vi "ValidateResults.vi"(8 "start_icfft":i32, 9 "PowerSpectrum":dbl[][](array[numeric]), 10 "Array of Power\nSpectrum Data":T1[](array[typedef]), 11 "Max Error":dbl) -> (2 "Boolean":bool, 3 "Max Error":dbl[](array[numeric]))   [LabVIEW 2015, in "SETI_LV.lvlib"]
uses:
  TypeDefs/Power Spectrum Data.ctl
  SETI_LV.lvlib
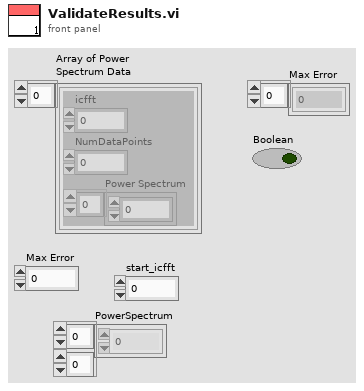
[diagram p1: front panel]
types:
  T1 = typedef "SETI_LV.lvlib/Power Spectrum Data.ctl" = cluster{"icfft":i32, "NumDataPoints":i32, "Power Spectrum":sgl[]}
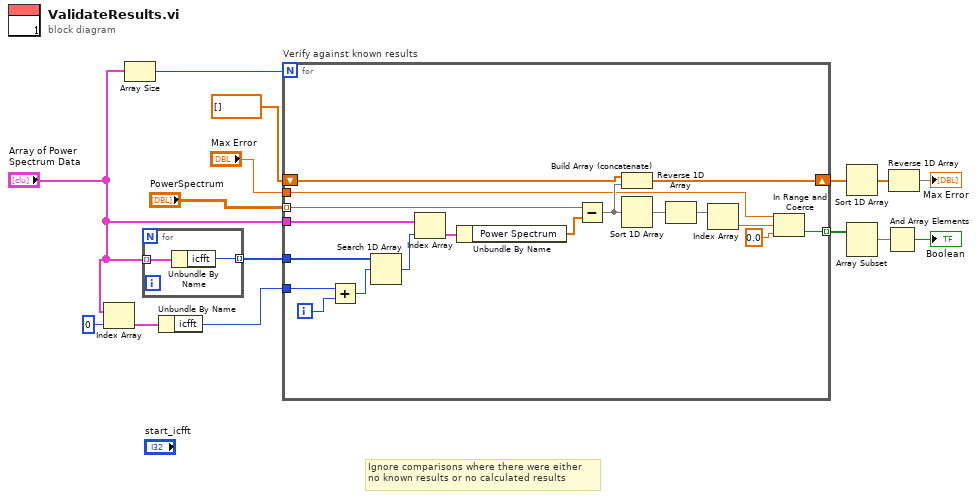
[diagram p0: block diagram]
diagram:
  # "Ignore comparisons where there were either\nno known results or no calculated results"
  n1 = Index Array(array="Array of Power\nSpectrum Data", index=0) -> (element=w2:T1)
  n2 = Array Size(array="Array of Power\nSpectrum Data") -> (size(s)=w5:i32)
  n3 = for {
    tunnel: "Array of Power\nSpectrum Data" -> [w17] mode=indexing
    tunnel: [w16] -> w9 mode=indexing
    n4 = Unbundle By Name(w17) -> ("icfft"=w16:i32)
  }
  n5 = Unbundle By Name(w2) -> ("icfft"=w1:i32)
  n6 = for "Verify against known results" {
    N: w5 -> [_]
    tunnel: "PowerSpectrum" -> [w23] mode=indexing
    tunnel: w1 -> [w34]
    tunnel: w9 -> [w31]
    tunnel: [w24] -> w10 mode=indexing
    tunnel: "Array of Power\nSpectrum Data" -> [w19]
    shift-right: [w21] -> w12
    shift-left: dbl[] [] -> [w20]
    tunnel: "Max Error" -> [w18]
    i -> [w33]
    n7 = Add(x=w34, y=w33) -> (x+y=w32:i32)
    n8 = Search 1D Array(1D array=w31, element=w32) -> (index of element=w35:i32)  [unwired: 1 in]
    n9 = Index Array(array=w19, index=w35) -> (element=w25:T1)
    n10 = Unbundle By Name(w25) -> ("Power Spectrum"=w27:sgl[])
    n11 = Subtract(x=w23, y=w27) -> (x-y=w22:dbl[])
    n12 = Build Array (concatenate)(w20, w22) -> (w21:dbl[])
    n13 = Sort 1D Array(array=w22) -> (sorted array=w26:dbl[])
    n14 = Reverse 1D Array(array=w26) -> (reversed array=w28:dbl[])
    n15 = Index Array(array=w28) -> (element=w30:dbl)  [unwired: 1 in]
    n16 = In Range and Coerce(upper limit=w18, x=w30, lower limit=0.0) -> (In Range?=w24:bool)  [unwired: 1 out]
  }
  n17 = Sort 1D Array(array=w12) -> (sorted array=w11:dbl[])
  n18 = Array Subset(array=w10) -> (w7:bool[])  [unwired: 2 in]
  n19 = And Array Elements(Boolean array=w7) -> (logical AND=→"Boolean":bool)
  n20 = Reverse 1D Array(array=w11) -> (reversed array=→"Max Error":dbl[])
